vi "LEDStateControl.vi"   [LabVIEW 2018]
uses:
  RobotStates.vi
  Inputs_DriverStation.vi
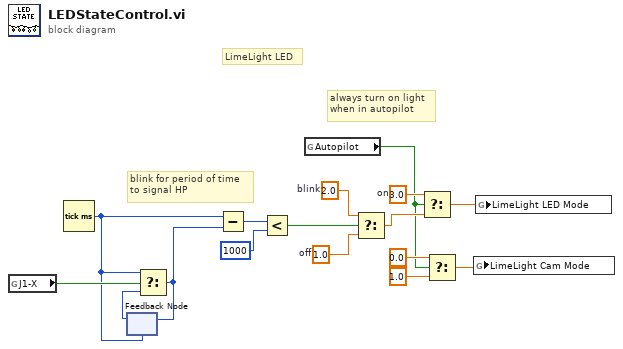
[diagram p0: block diagram]
diagram:
  w12 = 2.0  # blink
  w13 = 1.0  # off
  w15 = 3.0  # on
  # "LimeLight LED"
  # "always turn on light\nwhen in autopilot"
  # "blink for period of time\nto signal HP"
  n1 = global read "Inputs_DriverStation.vi" "J1-X"() -> (w11:bool)
  n2 = Tick Count (ms)() -> (millisecond timer value=w9:u32)
  n3 = feedback #1(w9) -> (w10:u32)
  n4 = Select(t=w9, s=w11, f=w10) -> (s? t:f=w8:u32)
  n5 = feedback-in #1(w8) -> ()
  n6 = Subtract(x=w9, y=w8) -> (x-y=w7:u32)
  n7 = Less?(x=w7, y=u32 1000) -> (x < y?=w5:bool)
  n8 = global read "RobotStates.vi" "Autopilot"() -> (w2:bool)
  n9 = Select(t=w12, s=w5, f=w13) -> (s? t:f=w14:dbl)
  n10 = Select(t=w15, s=w2, f=w14) -> (s? t:f=w16:dbl)
  n11 = Select(t=0.0, s=w2, f=1.0) -> (s? t:f=w1:dbl)
  n12 = global write "RobotStates.vi" "LimeLight Cam Mode"(w1) -> ()
  n13 = global write "RobotStates.vi" "LimeLight LED Mode"(w16) -> ()
